vi "Close Connection.vi"(8 "error in (no error)":errorcluster, 11 "NI-6537 (PXIe) in":refnum<class "NI-6537 (PXIe).lvclass">) -> (0 "error out":errorcluster, 3 "NI-6537 (PXIe) out":refnum<class "NI-6537 (PXIe).lvclass">)   [LabVIEW 2020, in "NI-6537 (PXIe).lvclass"]
uses:
  NI-6537 (PXIe).lvclass
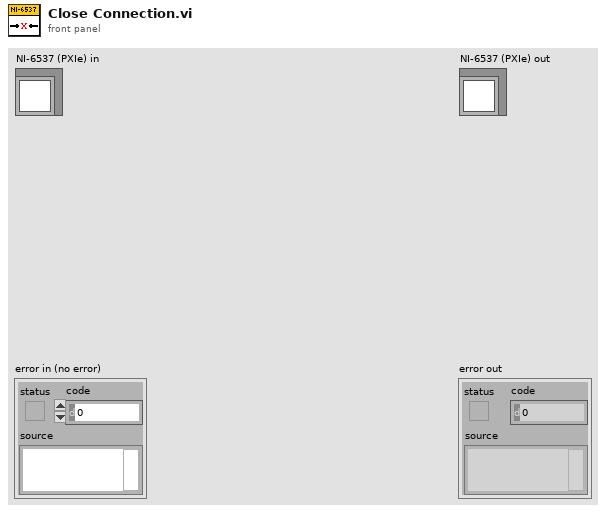
[diagram p1: front panel]
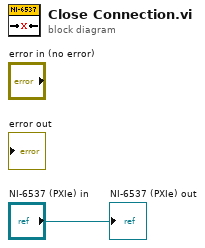
[diagram p0: block diagram]
diagram:
  "NI-6537 (PXIe) out" <- "NI-6537 (PXIe) in"
